vi "Draw Gate On XY Chart.vi"(6 "pen":T1={"Lable"="", "Visible"=FALSE, "Width"=2, "Colour"=16711680, "Line"=enum."DashDotDot"} {"Width" min=1 max=5}, 7 "Picture in":picture, 8 "error in (no error)":errorcluster, 10 "Inspection Gate":T2={"Start (us)"=2.0, "Length (us)"=7.0, "Threshold"=100, "Name"="", "Enabled?"=FALSE, "Colour"=0} {"Threshold" min=10 max=4095 step=10; "Length (us)" min=0.0 max=96000.0 step=100.0; "Start (us)" min=0.0 max=64000.0 step=100.0}, 11 "XY Graph":refnum<vi>) -> (0 "error out":errorcluster, 3 "Picture out":picture)   [LabVIEW 2026, in "MicroPulse_Driver.lvlib"]
uses:
  MicroPulse_Driver.lvlib
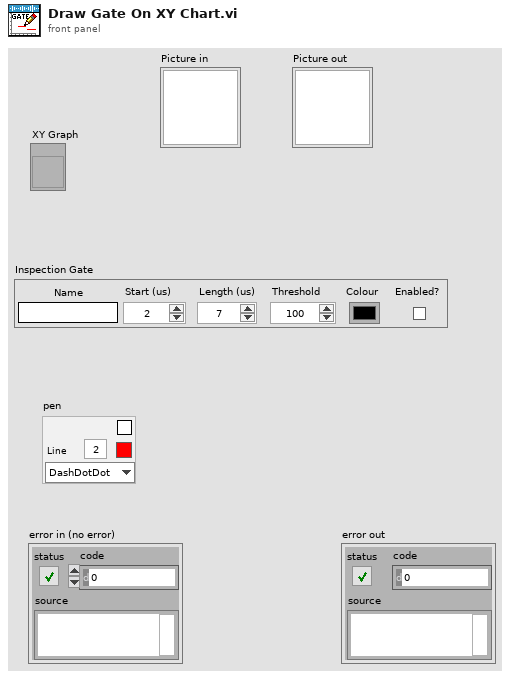
[diagram p1: front panel]
types:
  T1 = cluster{"Lable":string, "Visible":bool, "Width":u16, "Colour":u32, "Line":enum32{"Solid", "Dash", "Dot", "DashDot", "DashDotDot"}}
  T2 = cluster{"Start (us)":dbl, "Length (us)":dbl, "Threshold":u16, "Name":string, "Enabled?":bool, "Colour":u32}
  T3 = cluster{"horizontal":enum16{"left", "center", "right"}, "vertical":enum16{"top", "center", "bottom"}}
  T4 = typedef "LVRectTypeDef.ctl" = cluster{"Left":i16, "Top":i16, "Right":i16, "Bottom":i16}
  T5 = typedef "LVPoint32TypeDef.ctl" = cluster{"Horizontal":i32, "Vertical":i32}
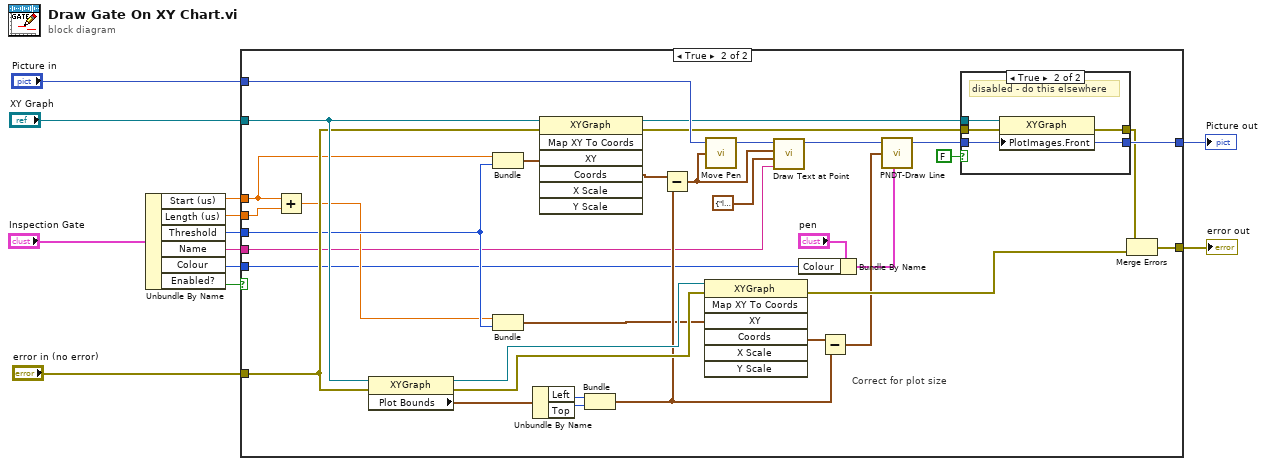
[diagram p0: block diagram]
diagram:
  n1 = Unbundle By Name("Inspection Gate") -> ("Start (us)"=w4:dbl, "Length (us)"=w6:dbl, "Threshold"=w5:u16, "Name"=w2:string, "Colour"=w1:u32, "Enabled?"=w3:bool)
  n2 = case shown="True" w3 {
    tunnel: "XY Graph" -> [_ w48]
    tunnel: [w13 w47] -> w10
    tunnel: "error in (no error)" -> [w13 w46]
    tunnel: [w14 w45] -> w8
    tunnel: "Picture in" -> [w14 w44]
    tunnel: w6 -> [_ w43]
    tunnel: w5 -> [_ w22]
    tunnel: w4 -> [_ w19]
    tunnel: w2 -> [_ w17]
    tunnel: w1 -> [_ w15]
    frame False {
    }
    frame True {
      # "Correct for plot size"
      n3 = Add(x=w19, y=w43) -> (x+y=w18:dbl)
      n4 = property on="Property Node" class="XYGraph"(reference=w48, error in=w46) -> (reference out=w41:refnum<vi>, error out=w42:errorcluster, "Plot Bounds"=w39:T4)
      n5 = Bundle("Start (us)"=w19, "Threshold"=w22) -> (w28:cluster{"Start (us)":dbl, "Threshold":u16})  [unwired: 1 in]
      n6 = Bundle(w18, "Threshold"=w22) -> (w26:cluster{dbl, "Threshold":u16})  [unwired: 1 in]
      n7 = Unbundle By Name(w39) -> ("Left"=w38:i16, "Top"=w37:i16)
      n8 = invoke class="XYGraph" method="Map XY To Coords"(reference=w48, error in=w46, "XY"=w28) -> (reference out=w33:refnum<vi>, error out=w32:errorcluster, "Coords"=w27:T5)  [unwired: 4 in, 4 out]
      n9 = Bundle("Left"=w38, "Top"=w37) -> (w40:cluster{"Left":i16, "Top":i16})  [unwired: 1 in]
      n10 = Subtract(x=w27, y=w40) -> (x-y=w31:T5)
      n11 = invoke class="XYGraph" method="Map XY To Coords"(reference=w41, error in=w42, "XY"=w26) -> (error out=w29:errorcluster, "Coords"=w25:T5)  [unwired: 4 in, 5 out]
      n12 = call <vilib>:"Move Pen.vi"("new position"=w31, "picture"=w44) -> ("new picture"=w34:picture)  [unwired: 1 in, 2 out]
      n13 = call <vilib>:"Draw Text at Point.vi"("text"=w17, "alignment(left, top)"=T3 {"horizontal"=enum."left", "vertical"=enum."bottom"}, "origin"=w31, "picture"=w34) -> ("new picture"=w35:picture)  [unwired: 6 in, 1 out]
      n14 = Bundle By Name(cluster="pen", "Colour"=w15) -> (w16:T1)
      n15 = Subtract(x=w25, y=w40) -> (x-y=w24:T5)
      n16 = call "PNDT-Draw Line.vi"("picture"=w35, "end point"=w24, "pen"=w16) -> ("new picture"=w20:picture)  [unwired: 6 in]
      n17 = case shown="True" FALSE {
        tunnel: w32 -> [w49 w54]
        tunnel: w33 -> [_ w53]
        tunnel: [w49 w52] -> w36
        tunnel: w20 -> [w50 w51]
        tunnel: [w50 w51] -> w45
        frame False {
        }
        frame True {
          # "disabled - do this elsewhere"
          n18 = property on="Property Node" class="XYGraph"(reference=w53, error in=w54, "PlotImages.Front"=w51) -> (error out=w52:errorcluster)  [unwired: 1 out]
        }
      }
      n19 = Merge Errors(w36, w29) -> (w47:errorcluster)
    }
  }
  "error out" <- w10
  "Picture out" <- w8
